vi "RIB Req - No Outputs.vi"(0 "Limits File Path":path, 5 "Results File Path":path, 11 "error in":errorcluster) -> (4 "Results Data Array":string[][](array[string]), 15 "error out":errorcluster)   [LabVIEW 2024]
doc: "Template test"
uses:
  <vilib>/addons/_JKI Toolkits/State Machine/_JKI_lib_State_Machine.llb/Select State(s)_err__jki_lib_state_machine.vi
  <vilib>/DAQmx/read.llb/DAQmx Read (Digital 1D Bool 1Chan 1Samp).vi
  <vilib>/addons/_JKI Toolkits/State Machine/_JKI_lib_State_Machine.llb/Select State(s)_bool__jki_lib_state_machine.vi
  <vilib>/addons/_JKI Toolkits/State Machine/_JKI_lib_State_Machine.llb/Periodic Trigger__ogtk__JKI-SM__jki_lib_state_machine.vi
  <userlib>/_OpenG.lib/file/file.llb/Strip Path Extension - String__ogtk.vi
  <vilib>/Utility/file.llb/Read Delimited Spreadsheet (string).vi
  <vilib>/DAQmx/miscellaneous.llb/DAQmx Fill In Error Info.vi
  <userlib>/_OpenG.lib/file/file.llb/openg_file.lvlib
  <userlib>/_OpenG.lib/appcontrol/appcontrol.llb/openg_application_control.lvlib
  <userlib>/_OpenG.lib/time/time.llb/openg_time.lvlib
  <vilib>/Utility/file.llb/Write Delimited Spreadsheet (string).vi
panel:
  in  "False":bool
  out "Results Data 3":string[](array[string])
  in  "task out":refnum<k21>
  out "Timeout":dbl(slide) scale=0.0..5.0
  in  "Exit":bool
  # "Both 15A and 5A Outputs are False"
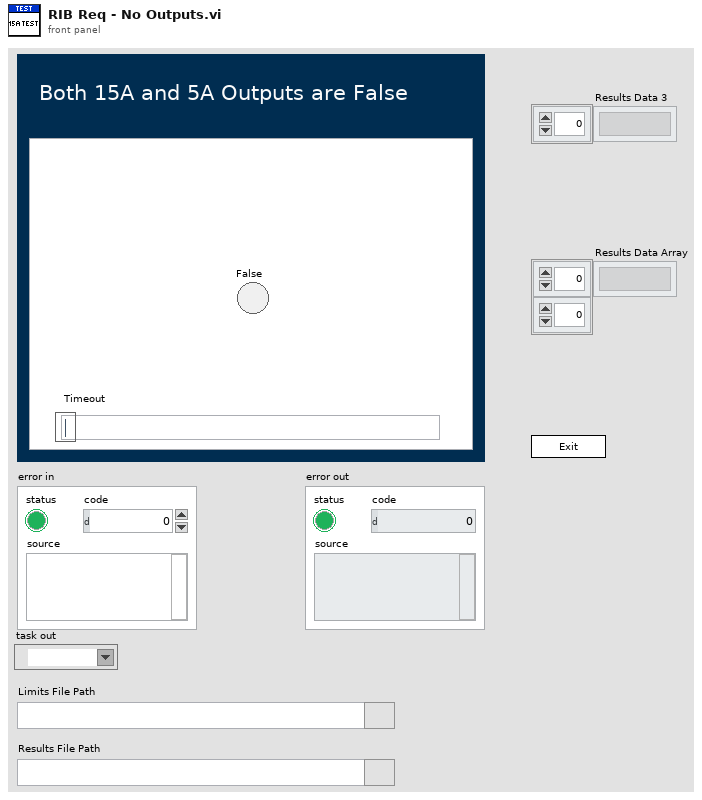
[diagram p1: front panel]
types:
  T1 = enum32{"Invalid", "Standard", "Closed", "Hidden", "Minimized", "Maximized"}
  T2 = enum32{"invalid app kind", "Development System", "Run Time System", "Student Edition", "Embedded LabVIEW", "Evaluation", "Custom"}
  T3 = typedef "FGV - Enum" = enum16{"Cleanup", "Get Data", "Simulator", "Open UDP", "Initialise DAQ", "Initialise I2C"}
  T4 = enum16{"Start Timer", "Get Time", "Pause", "Unpause"}
  T5 = cluster{"Core":cluster{"Current VI Reference":refnum<vi>, "Close Panel on Exit?":bool}, "Limits File Path":path, "Test Limits":string[][], "Results Data Array":string[][], "Results File Path":path, "task out":refnum<k21>, "False":bool}
  T6 = cluster{"Current VI Reference":refnum<vi>, "Close Panel on Exit?":bool}
  T7 = cluster{"[0]":bool, "[1]":bool, "[2]":bool, "[3]":bool, "[4]":bool, "[5]":bool, "[6]":bool, "[7]":bool, "[8]":bool}
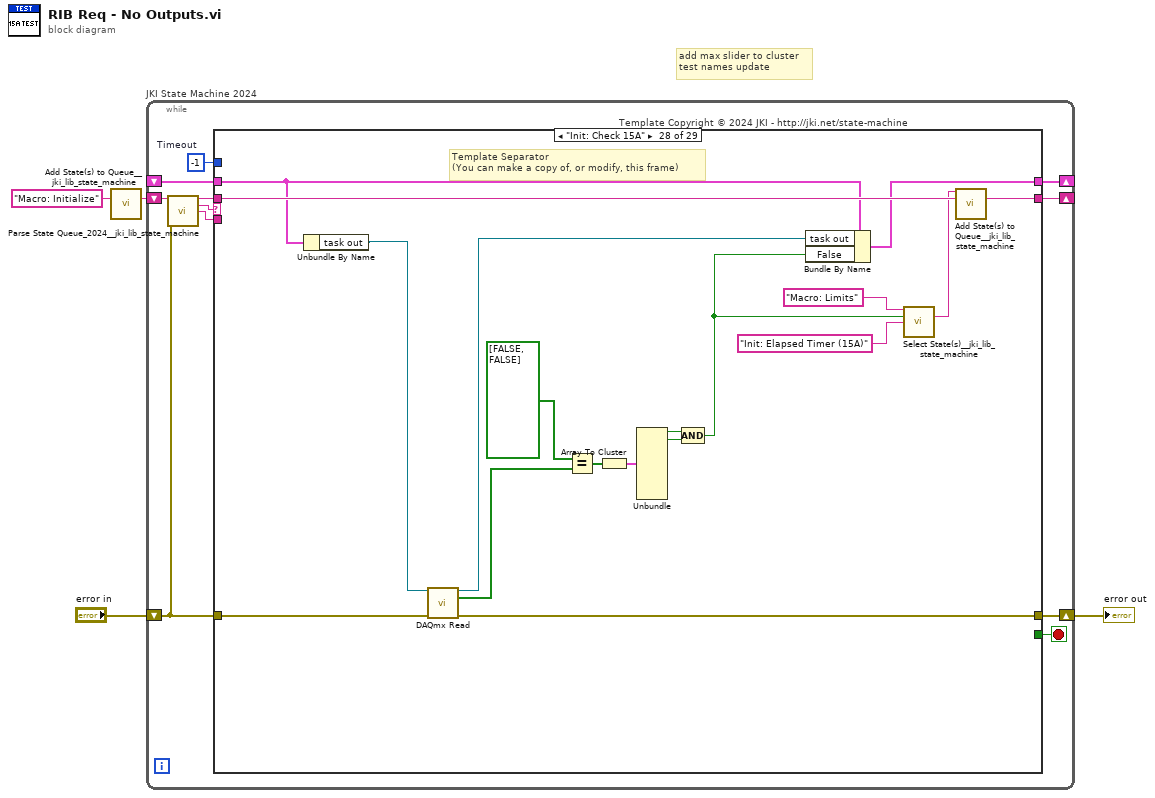
[diagram p0: block diagram]
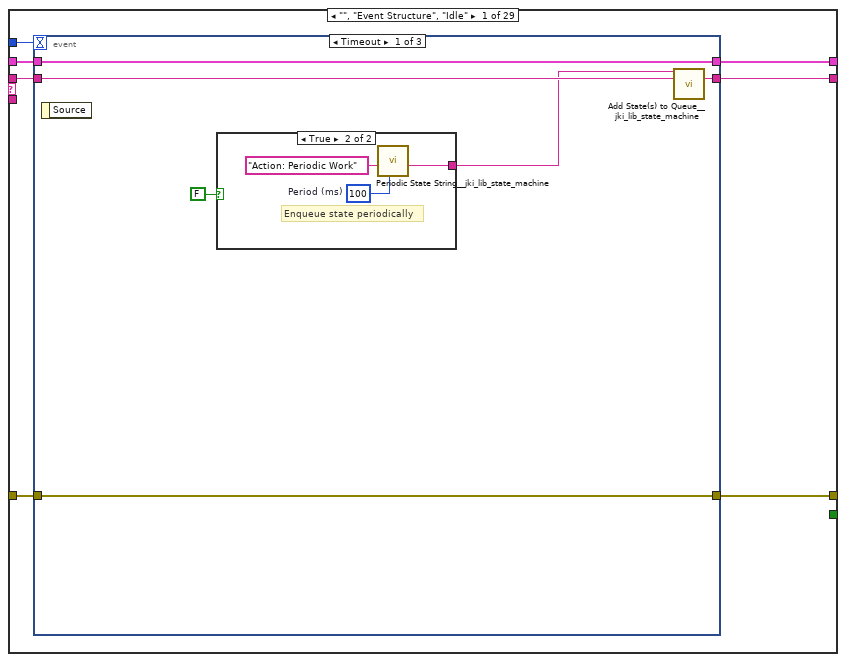
[diagram p2: hidden frame]
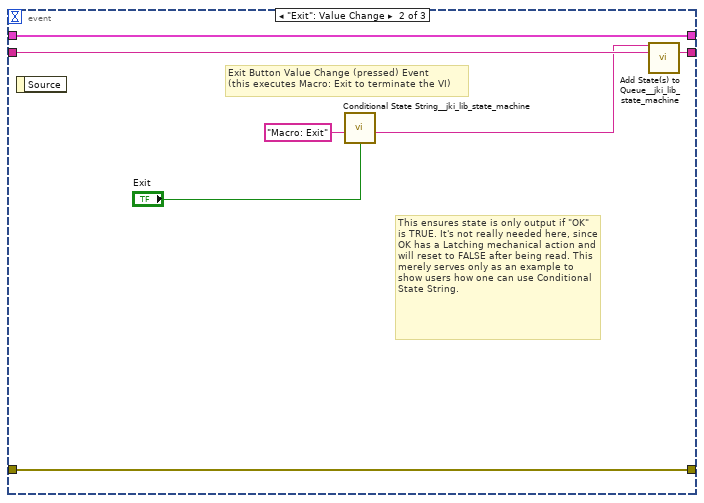
[diagram p4: hidden frame]
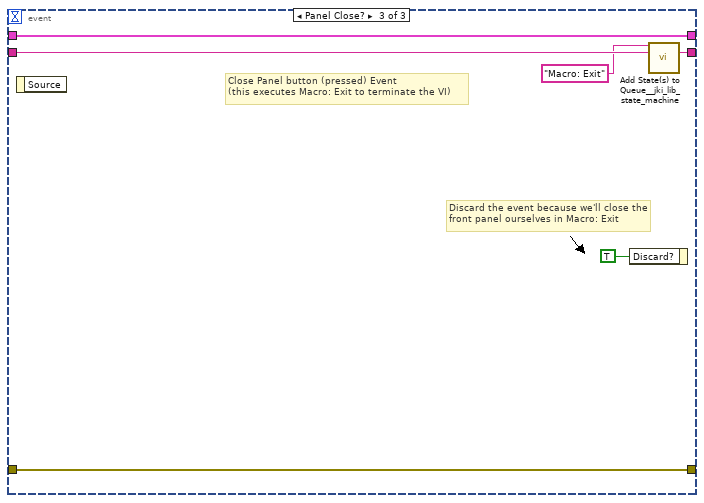
[diagram p5: hidden frame]
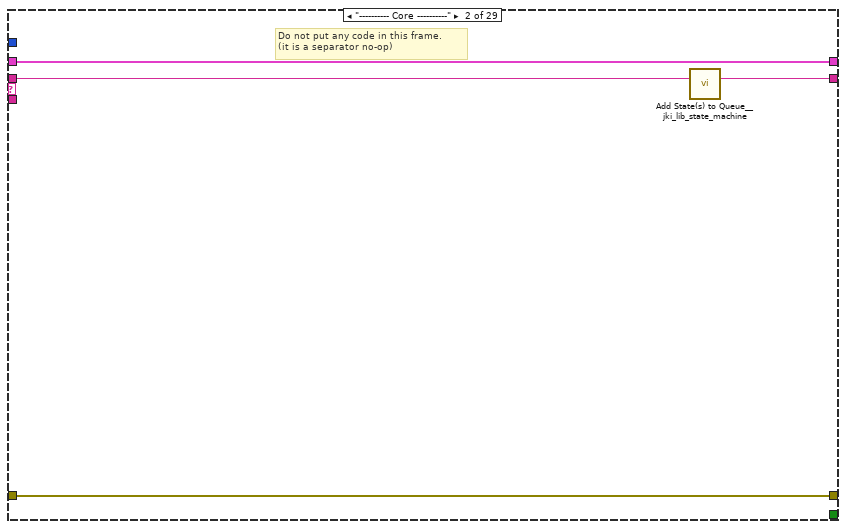
[diagram p6: hidden frame]
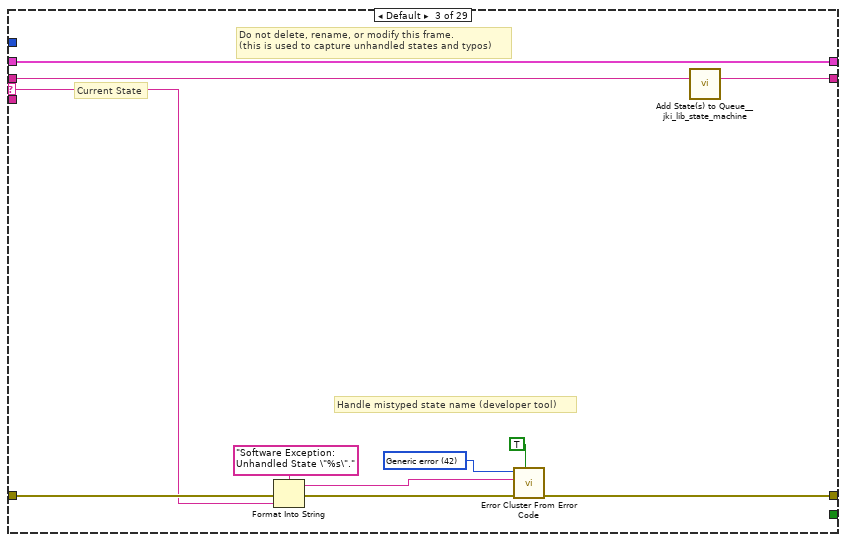
[diagram p7: hidden frame]
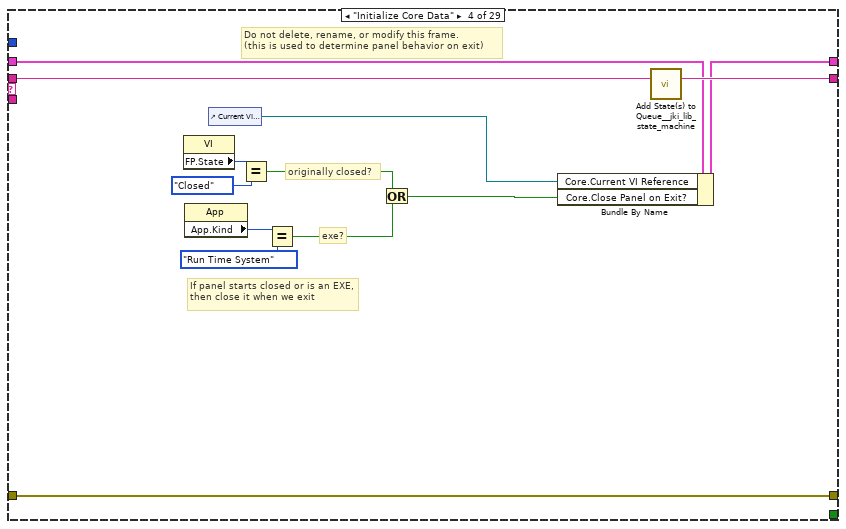
[diagram p8: hidden frame]
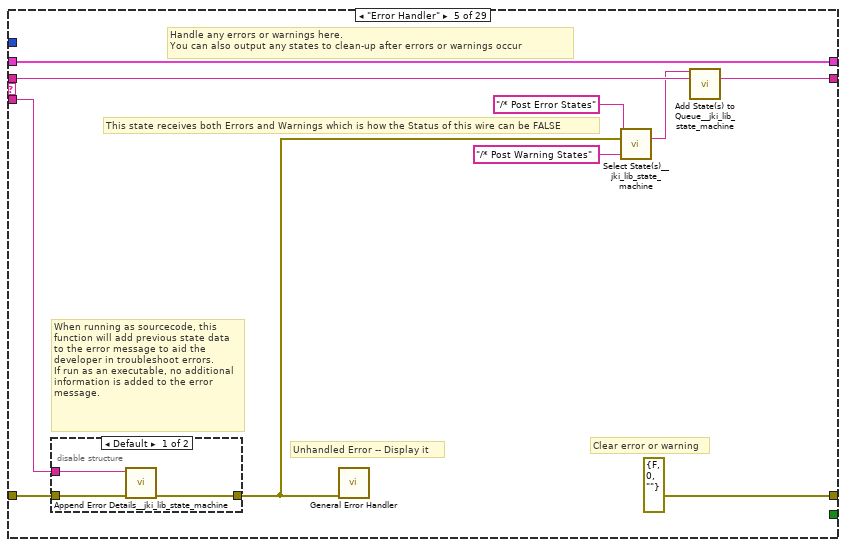
[diagram p9: hidden frame]
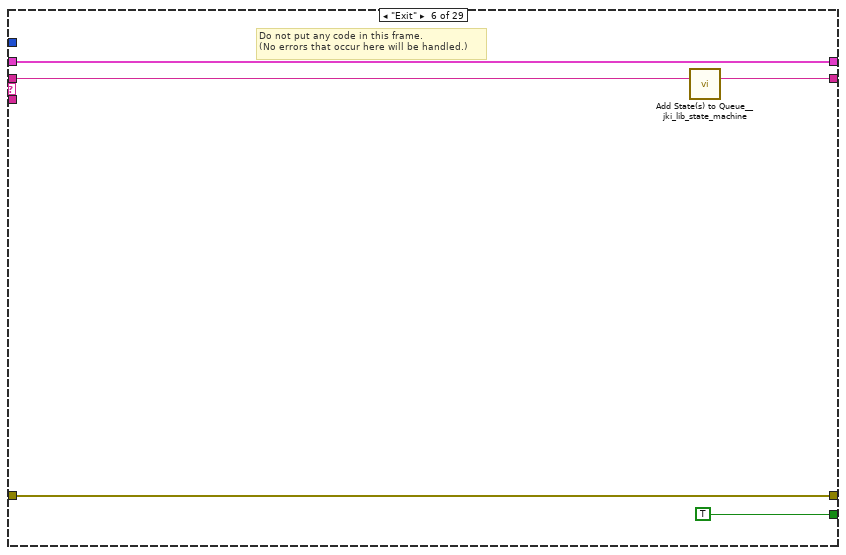
[diagram p11: hidden frame]
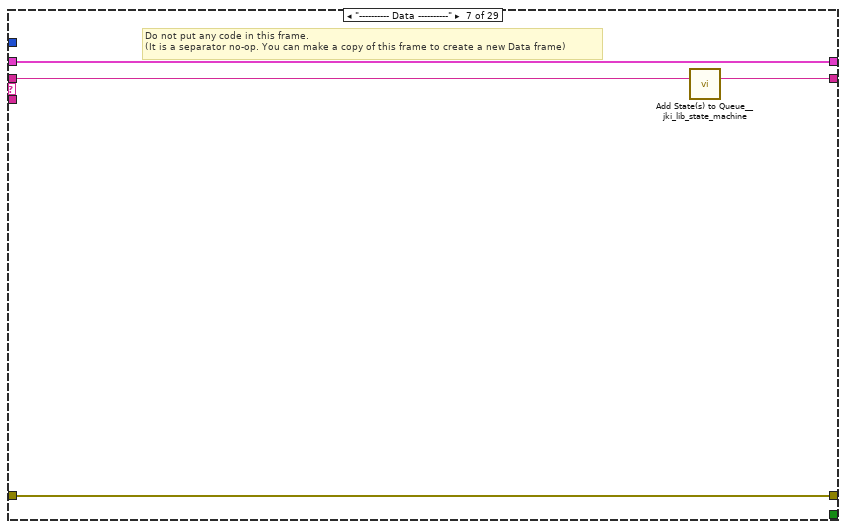
[diagram p12: hidden frame]
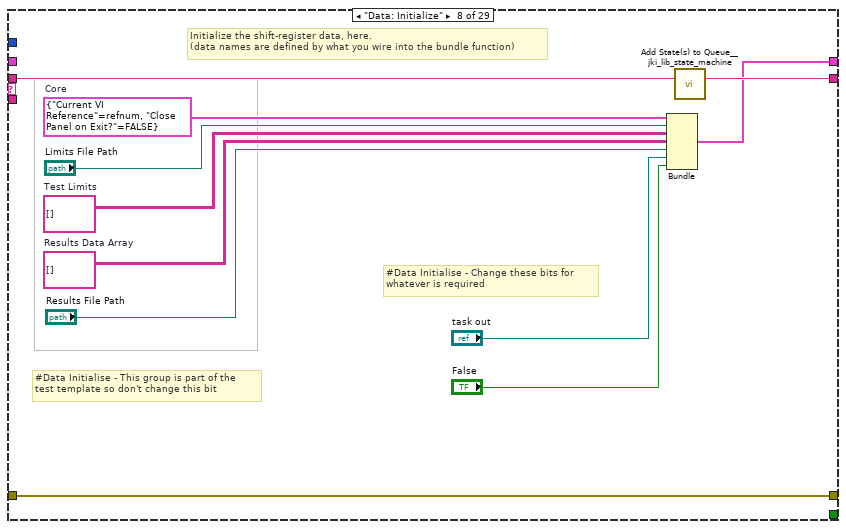
[diagram p13: hidden frame]
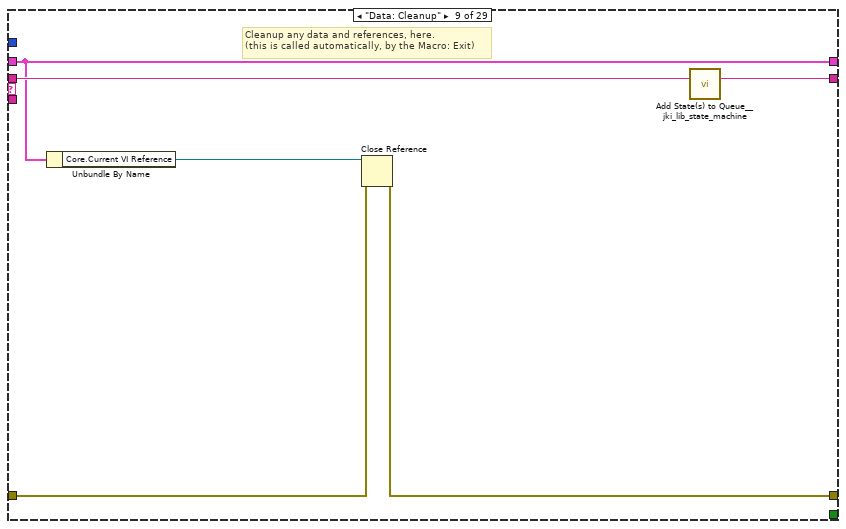
[diagram p14: hidden frame]
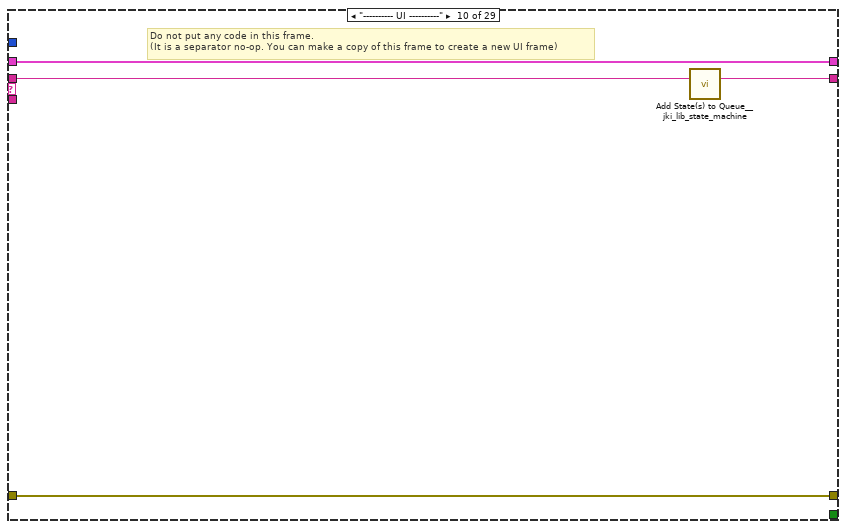
[diagram p15: hidden frame]
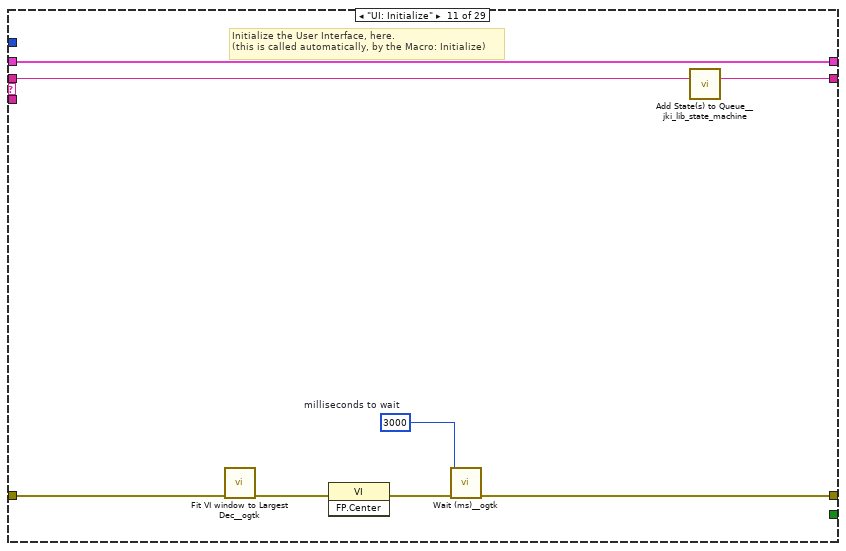
[diagram p16: hidden frame]
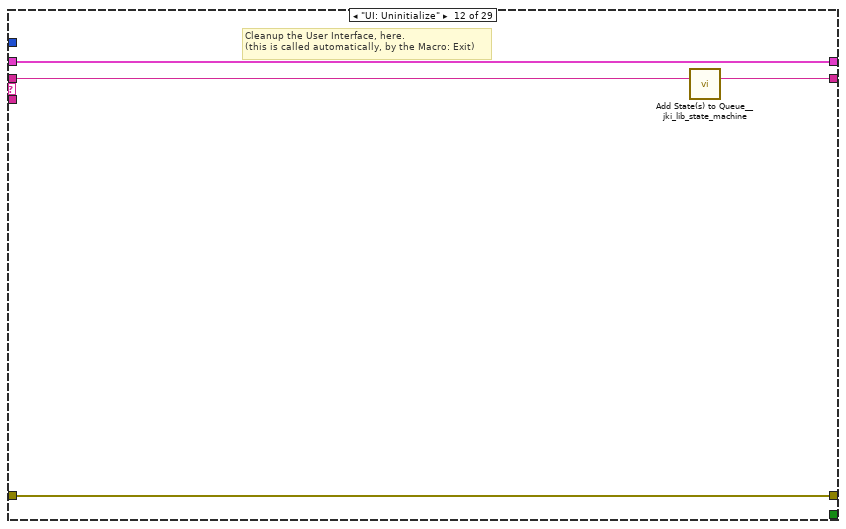
[diagram p17: hidden frame]
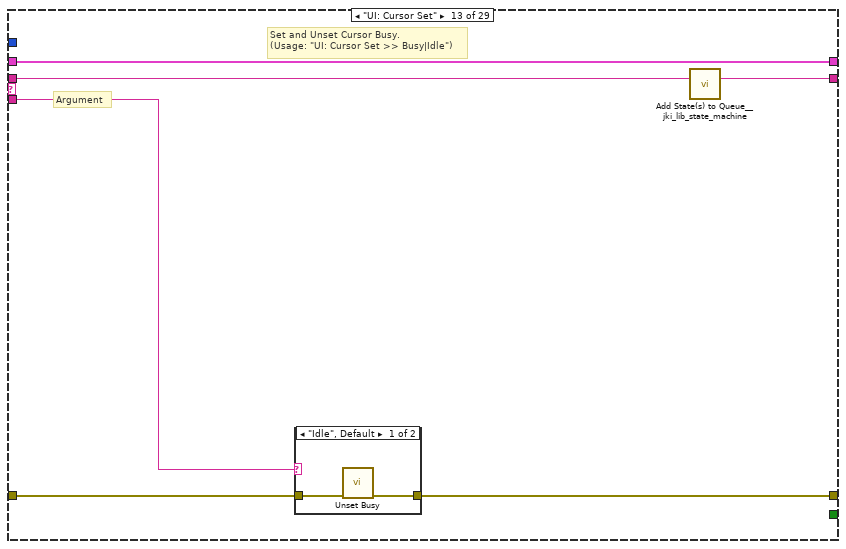
[diagram p18: hidden frame]
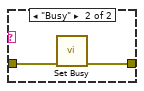
[diagram p19: hidden frame]
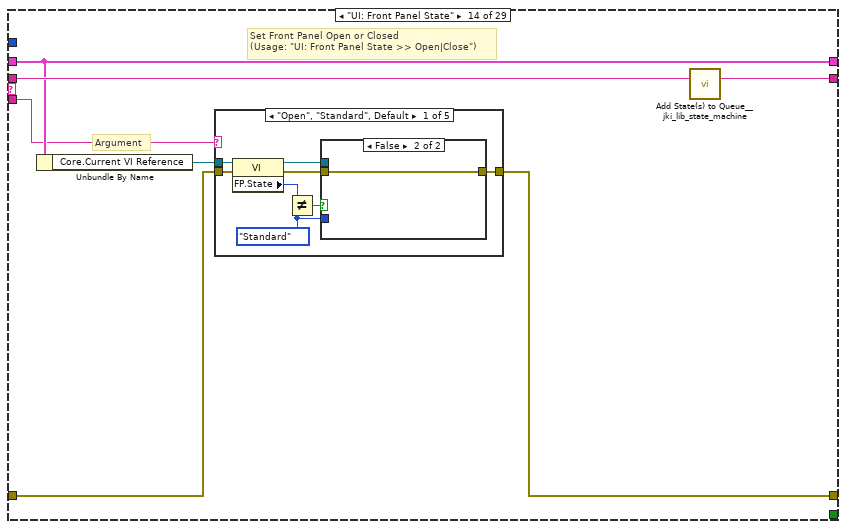
[diagram p20: hidden frame]
diagram:
  # "add max slider to cluster \ntest names update"
  n1 = call <vilib>:"Add State(s) to Queue__jki_lib_state_machine.vi"("State(s) in (\"\")"="Macro: Initialize") -> ("States Out"=w4:string)  [unwired: 14 in]
  n2 = while "JKI State Machine 2024" {
    shift-right: [w8] -> _
    shift-left: _ -> [w7]
    shift-right: [w11] -> w1
    shift-left: "error in" -> [w5]
    shift-right: [w10] -> _
    shift-left: w4 -> [w12]
    stop <- w9 stop-if-true
    w6 = -1  # Timeout
    # "Template Copyright © 2024 JKI - http://jki.net/state-machine"
    n3 = call <vilib>:"Parse State Queue_2024__jki_lib_state_machine.vi"("State Queue"=w12, "Error In (no error)"=w5) -> ("Remaining States"=w14:string, "Current State"=w15:string, "Arguments"=w13:string)  [unwired: 11 in]
    n4 = case shown="\"Init: Check 15A\"" w15 {
      selector: w15 -> [_ _ w49 _ _ _ _ _ _ _ _ _ _ _ _ _ _ _ _ _ _ _ _ _ _ _ _ _ _]
      tunnel: w14 -> [w22 w48 w53 w72 w82 w91 w95 w106 w112 w116 w124 w128 w134 w145 w214 w219 w224 w229 w238 w242 w255 w272 w276 w285 w289 w297 w308 w326 w338]
      tunnel: w13 -> [_ _ _ _ w77 _ _ _ _ _ _ _ w129 w139 _ _ _ _ _ _ _ _ _ _ _ _ _ _ _]
      tunnel: w7 -> [w20 w45 w51 w65 w79 w89 w92 _ w107 w113 w122 w126 w132 w141 w211 w216 w221 w226 w236 w239 w245 w264 w273 w281 w286 w295 w306 w322 w336]
      tunnel: [w19 w46 w55 w69 errorcluster {"status"=FALSE, "code"=0, "source"=""} ("error out") w88 w93 w103 w108 w114 w120 w125 w130 w142 w212 w217 w222 w227 w233 w240 w251 w269 w274 w283 w287 w292 w301 w312 w333] -> w11
      tunnel: w5 -> [w16 w46 w54 w69 w78 w88 w93 w103 w109 w114 w121 w125 w131 w143 w212 w217 w222 w227 w233 w240 w250 w268 w274 w282 w287 w291 w304 w313 w334]
      tunnel: [w21 w47 w52 w71 w81 w90 w94 w105 w111 w115 w123 w127 w133 w144 w213 w218 w223 w228 w237 w241 w254 w271 w275 w284 w288 w296 w307 w325 w337] -> w10
      tunnel: [_ _ _ _ _ TRUE _ _ _ _ _ _ _ _ _ _ _ _ _ _ _ _ _ _ _ _ _ _ _] -> w9
      tunnel: [w18 w45 w51 w70 w79 w89 w92 w104 w107 w113 w122 w126 w132 w141 w211 w216 w221 w226 w236 w239 w244 w263 w273 w281 w286 w294 w306 w321 w336] -> w8
      tunnel: w6 -> [w17 _ _ _ _ _ _ _ _ _ _ _ _ _ _ _ _ _ _ _ _ _ _ _ _ _ _ _ _]
      frame "", "Event Structure", "Idle" {
        n5 = event shown="[0] Timeout" {
          selector: _ -> [_ _ _]
          dyn-events: _ -> [_ _ _]
          timeout: w17 -> [_ _ _]
          tunnel: w22 -> [w28 w38 w44]
          tunnel: [w27 w37 w43] -> w21
          tunnel: w20 -> [w25 w35 w41]
          tunnel: [w26 w36 w42] -> w19
          tunnel: w16 -> [w26 w36 w42]
          tunnel: [w25 w35 w41] -> w18
          event Timeout {
            n6 = event-data() -> ()  [unwired: 1 in, 1 out]
            n7 = case shown="True" FALSE {
              tunnel: [_ w31] -> w24
              frame False {
              }
              frame True {
                w29 = u32 100  # Period (ms)
                # "Enqueue state periodically"
                n8 = call <vilib>:"Periodic State String__jki_lib_state_machine.vi"("Period (ms)"=w29, "State"="Action: Periodic Work") -> ("State Out"=w31:string)  [unwired: 9 in]
              }
            }
            n9 = call <vilib>:"Add State(s) to Queue__jki_lib_state_machine.vi"("State(s) in Front (\"\")"=w24, "State(s) in (\"\")"=w28) -> ("States Out"=w27:string)  [unwired: 13 in]
          }
          event "Exit": Value Change {
            # "This ensures state is only output if \"OK\" is TRUE. It's not really needed here, since OK has a Latching mechanical action and will reset to FALSE after being read. This merely serves only as an example to show users how one can use Conditional State String."
            # "Exit Button Value Change (pressed) Event\n(this executes Macro: Exit to terminate the VI)"
            n10 = event-data() -> ()  [unwired: 1 in, 1 out]
            n11 = call <vilib>:"Conditional State String__jki_lib_state_machine.vi"("Do State(s)?"="Exit", "State"="Macro: Exit") -> ("State Out"=w32:string)  [unwired: 7 in]
            n12 = call <vilib>:"Add State(s) to Queue__jki_lib_state_machine.vi"("State(s) in Front (\"\")"=w32, "State(s) in (\"\")"=w38) -> ("States Out"=w37:string)  [unwired: 13 in]
          }
          event Panel Close? {
            # "Discard the event because we'll close the front panel ourselves in Macro: Exit"
            # "Close Panel button (pressed) Event\n(this executes Macro: Exit to terminate the VI)"
            n13 = event-data() -> ()  [unwired: 1 in, 1 out]
            n14 = event-data("Discard?"=TRUE) -> ()  [unwired: 1 in, 1 out]
            n15 = call <vilib>:"Add State(s) to Queue__jki_lib_state_machine.vi"("State(s) in Front (\"\")"="Macro: Exit", "State(s) in (\"\")"=w44) -> ("States Out"=w43:string)  [unwired: 13 in]
          }
        }
      }
      frame "---------- Core ----------" {
        # "Do not put any code in this frame.\n(it is a separator no-op)"
        n16 = call <vilib>:"Add State(s) to Queue__jki_lib_state_machine.vi"("State(s) in (\"\")"=w48) -> ("States Out"=w47:string)  [unwired: 14 in]
      }
      frame Default {
        w58 = 42 items=["No error", "Argument error", "Memory is full", "Out of zone", "End of file", "File already open", "Generic file I/O error", "File not found", "File permission error", "Disk is full", "Duplicate path", "Too many files open", "System feature not enabled", "Resource file not found", "Cannot add resource", "Resource not found", "Image not found", "Image memory error", "Pen does not exist", "Config type invalid", "Config token not found", "Config parse error", "Config memory error", "Bad external code format", "Bad external code offset", "External code not present", "Null window", "Destroy window error", "Null menu", "Print aborted", "Bad print record", "Print driver error", "Windows error during printing", "Memory error during printing", "Print dialog error", "Generic print error", "Invalid device refnum", "Device not found", "Device parameter error", "Device unit error", "Cannot open device", "Device call aborted", "Generic error", "Cancelled by user", "Object ID too low", "Object ID too high", "Object not in heap", "Unknown heap", "Unknown object (invalid DefProc)", "Unknown object (DefProc not in table)", "Message out of range", "Invalid (null) method", "Unknown message", "Manager call not supported", "Bad address", "Network operation in progress", "Network operation timed out", "Connection is busy", "Network attribute not supported", "Network error", "Address in use", "System out of memory", "Connection aborted", "Connection refused", "Not connected", "Already connected", "Connection closed", "Initialization error (interapplication manager)", "Bad occurrence", "Wait on unbound occurrence handler", "Occurrence queue overflow", "Datalog type conflict", "Unused", "Unrecognized type (interapplication manager)", "Memory corrupt", "Failed to make temporary DLL", "Old CIN version", "Drag socket not found", "Failed to load drop-object", "Failed to register OLE object", "Failed to release OLE object", "Format specifier type mismatch", "Unknown format specifier", "Too few format specifiers", "Too many format specifiers", "Scan failed", "Newer CIN version", "Error converting to variant", "Runtime menu error", "Password tampered", "Variant attribute not found", "Incompatible variant data type", "Event data is not available", "Event Store is not present", "Occurrence is not found", "Event Queue is not created", "Event info is not available", "Refnum passed is NULL", "Error retrieving Class GUID", "Error retrieving CoClass GUID", "Error retrieving TypeLib GUID.", "Bad built application magic bytes.", "Specific driver is different from the specific driver associated with the Logical Name.", "There is no session opened to the class driver.", "Max Error", "MAX - Error with config objects", "MAX - Error loading configuration", "MAX - Group not supported"]
        # "Current State"
        # "Do not delete, rename, or modify this frame.\n(this is used to capture unhandled states and typos)"
        # "Handle mistyped state name (developer tool)"
        n17 = Format Into String(format string="Software Exception: Unhandled State \"%s\"." ("message"), error in=w54, w49) -> (resulting string=w57:string, error out=w56:errorcluster)  [unwired: 1 in]
        n18 = call <vilib>:"Error Cluster From Error Code.vi"("show call chain? (False)"=TRUE, "error in (no error)"=w56, "error message (\"\")"=w57, "error code (0)"=w58) -> ("error out"=w55:errorcluster)  [unwired: 5 in]
        n19 = call <vilib>:"Add State(s) to Queue__jki_lib_state_machine.vi"("State(s) in (\"\")"=w53) -> ("States Out"=w52:string)  [unwired: 14 in]
      }
      frame "Initialize Core Data" {
        # "Do not delete, rename, or modify this frame.\n(this is used to determine panel behavior on exit)"
        # "originally closed?"
        # "exe?"
        # "If panel starts closed or is an EXE, then close it when we exit"
        n20 = property class="VI"() -> ("FP.State"=w62:T1)  [unwired: 2 in, 2 out]
        n21 = property class="App"() -> ("App.Kind"=w68:T2)  [unwired: 2 in, 2 out]
        n22 = control-ref of="Current VI Reference"() -> (w63:refnum<vi>)
        n23 = Equal?(x=w62, y=T1."Closed" ("Front Panel Window:State")) -> (x = y?=w60:bool)
        n24 = Equal?(x=w68, y=T2."Run Time System" ("Application:Kind")) -> (x = y?=w66:bool)
        n25 = Or(x=w60, y=w66) -> (x .or. y?=w64:bool)
        n26 = Bundle By Name(cluster=w65, "Core.Current VI Reference"=w63, "Core.Close Panel on Exit?"=w64) -> (w70:T5)
        n27 = call <vilib>:"Add State(s) to Queue__jki_lib_state_machine.vi"("State(s) in (\"\")"=w72) -> ("States Out"=w71:string)  [unwired: 14 in]
      }
      frame "Error Handler" {
        # "When running as sourcecode, this function will add previous state data to the error message to aid the developer in troubleshoot errors.\nIf run as an executable, no additional information is added to the error message."
        # "This state receives both Errors and Warnings which is how the Status of this wire can be FALSE"
        # "Unhandled Error -- Display it"
        # "Handle any errors or warnings here.\nYou can also output any states to clean-up after errors or warnings occur"
        # "Clear error or warning"
        n28 = disable-structure shown="Default" {
          disable-tunnel: w78 -> [w85 w86]
          disable-tunnel: w77 -> [w84 _]
          disable-tunnel: [w83 w86] -> w76
          frame condition #0 (active) {
            n29 = call <vilib>:"Append Error Details__jki_lib_state_machine.vi"("error in (no error)"=w85, "Previous State and Argument(s)"=w84) -> ("error out"=w83:errorcluster)  [unwired: 9 in]
          }
          frame condition #1 {
          }
        }
        n30 = call <vilib>:"General Error Handler.vi"("error in (no error)"=w76) -> ()  [unwired: 10 in, 5 out]
        n31 = call-poly <vilib>:"Select State(s)__jki_lib_state_machine.vi"("State(s) if True (\"\")"="/* Post Error States", "Select"=w76, "State(s) if False (\"\")"="/* Post Warning States") -> ("States Out"=w74:string)  [unwired: 12 in]
        n32 = call <vilib>:"Add State(s) to Queue__jki_lib_state_machine.vi"("State(s) in Front (\"\")"=w74, "State(s) in (\"\")"=w82) -> ("States Out"=w81:string)  [unwired: 13 in]
      }
      frame "Exit" {
        # "Do not put any code in this frame.\n(No errors that occur here will be handled.)"
        n33 = call <vilib>:"Add State(s) to Queue__jki_lib_state_machine.vi"("State(s) in (\"\")"=w91) -> ("States Out"=w90:string)  [unwired: 14 in]
      }
      frame "---------- Data ----------" {
        # "Do not put any code in this frame.\n(It is a separator no-op. You can make a copy of this frame to create a new Data frame)"
        n34 = call <vilib>:"Add State(s) to Queue__jki_lib_state_machine.vi"("State(s) in (\"\")"=w95) -> ("States Out"=w94:string)  [unwired: 14 in]
      }
      frame "Data: Initialize" {
        w99 = string[][] []  # Results Data Array
        w100 = string[][] []  # Test Limits
        w102 = T6 {"Current VI Reference"=refnum, "Close Panel on Exit?"=FALSE}  # Core
        # "#Data Initialise - Change these bits for\nwhatever is required"
        # "#Data Initialise - This group is part of the\ntest template so don't change this bit"
        # "Initialize the shift-register data, here.\n(data names are defined by what you wire into the bundle function)"
        n35 = Bundle("Core"=w102, "Limits File Path"="Limits File Path", "Test Limits"=w100, "Results Data Array"=w99, "Results File Path"="Results File Path", "task out"="task out", "False"="False") -> (w104:T5)  [unwired: 1 in]
        n36 = call <vilib>:"Add State(s) to Queue__jki_lib_state_machine.vi"("State(s) in (\"\")"=w106) -> ("States Out"=w105:string)  [unwired: 14 in]
      }
      frame "Data: Cleanup" {
        # "Cleanup any data and references, here.\n(this is called automatically, by the Macro: Exit)"
        n37 = Unbundle By Name(w107) -> ("Core.Current VI Reference"=w110:refnum<vi>)
        n38 = Close Reference(reference=w110, error in (no error)=w109) -> (error out=w108:errorcluster)
        n39 = call <vilib>:"Add State(s) to Queue__jki_lib_state_machine.vi"("State(s) in (\"\")"=w112) -> ("States Out"=w111:string)  [unwired: 14 in]
      }
      frame "---------- UI ----------" {
        # "Do not put any code in this frame.\n(It is a separator no-op. You can make a copy of this frame to create a new UI frame)"
        n40 = call <vilib>:"Add State(s) to Queue__jki_lib_state_machine.vi"("State(s) in (\"\")"=w116) -> ("States Out"=w115:string)  [unwired: 14 in]
      }
      frame "UI: Initialize" {
        w119 = u32 3000  # milliseconds to wait
        # "Initialize the User Interface, here.\n(this is called automatically, by the Macro: Initialize)"
        n41 = call <userlib>:"Fit VI window to Largest Dec__ogtk.vi"("error in (no error)"=w121) -> ("error out"=w117:errorcluster)  [unwired: 5 in, 1 out]
        n42 = invoke class="VI" method="FP.Center"(error in=w117) -> (error out=w118:errorcluster)  [unwired: 2 in, 2 out]
        n43 = call <userlib>:"Wait (ms)__ogtk.vi"("error in (no error)"=w118, "milliseconds to wait"=w119) -> ("error out"=w120:errorcluster)  [unwired: 8 in, 1 out]
        n44 = call <vilib>:"Add State(s) to Queue__jki_lib_state_machine.vi"("State(s) in (\"\")"=w124) -> ("States Out"=w123:string)  [unwired: 14 in]
      }
      frame "UI: Uninitialize" {
        # "Cleanup the User Interface, here.\n(this is called automatically, by the Macro: Exit)"
        n45 = call <vilib>:"Add State(s) to Queue__jki_lib_state_machine.vi"("State(s) in (\"\")"=w128) -> ("States Out"=w127:string)  [unwired: 14 in]
      }
      frame "UI: Cursor Set" {
        # "Argument"
        # "Set and Unset Cursor Busy.\n(Usage: \"UI: Cursor Set >> Busy|Idle\")"
        n46 = case shown="\"Idle\", Default" w129 {
          tunnel: w131 -> [w136 w138]
          tunnel: [w135 w137] -> w130
          frame "Idle", Default {
            n47 = call <vilib>:"Unset Busy.vi"("error in (no error)"=w136) -> ("error out"=w135:errorcluster)  [unwired: 10 in]
          }
          frame "Busy" {
            n48 = call <vilib>:"Set Busy.vi"("error in (no error)"=w138) -> ("error out"=w137:errorcluster)  [unwired: 9 in, 1 out]
          }
        }
        n49 = call <vilib>:"Add State(s) to Queue__jki_lib_state_machine.vi"("State(s) in (\"\")"=w134) -> ("States Out"=w133:string)  [unwired: 14 in]
      }
      frame "UI: Front Panel State" {
        # "Argument"
        # "Set Front Panel Open or Closed\n(Usage: \"UI: Front Panel State >> Open|Close\")"
        n50 = Unbundle By Name(w141) -> ("Core.Current VI Reference"=w140:refnum<vi>)
        n51 = case shown="\"Open\", \"Standard\", Default" w139 {
          tunnel: w143 -> [w151 w166 w177 w190 w203]
          tunnel: [w153 w167 w179 w192 w205] -> w142
          tunnel: w140 -> [w152 w164 w178 w191 w204]
          frame "Open", "Standard", Default {
            w146 = T1."Standard" ("State")
            n52 = property class="VI"(reference=w152, error in=w151) -> (reference out=w149:refnum<vi>, error out=w150:errorcluster, "FP.State"=w148:T1)
            n53 = Not Equal?(x=w148, y=w146) -> (x != y?=w147:bool)
            n54 = case shown="False" w147 {
              tunnel: [w157 w159] -> w153
              tunnel: w150 -> [w156 w159]
              tunnel: w149 -> [w155 _]
              tunnel: w146 -> [w154 _]
              frame True {
                n55 = invoke class="VI" method="FP.Open"(reference=w155, error in=w156, "Activate"=TRUE, "State"=w154) -> (error out=w157:errorcluster)  [unwired: 1 in, 4 out]
              }
              frame False {
              }
            }
          }
          frame "Close", "Closed" {
            n56 = property class="VI"(reference=w164, error in=w166) -> (reference out=w163:refnum<vi>, error out=w165:errorcluster, "FP.State"=w161:T1)
            n57 = Not Equal?(x=w161, y=T1."Closed" ("Front Panel Window:State")) -> (x != y?=w160:bool)
            n58 = case shown="True" w160 {
              tunnel: [w168 w171] -> w167
              tunnel: w165 -> [w168 w170]
              tunnel: w163 -> [_ w169]
              frame False {
              }
              frame True {
                n59 = invoke class="VI" method="FP.Close"(reference=w169, error in=w170) -> (error out=w171:errorcluster)  [unwired: 1 in, 2 out]
              }
            }
          }
          frame "Hidden", "Hide" {
            w172 = T1."Hidden" ("State")
            n60 = property class="VI"(reference=w178, error in=w177) -> (reference out=w175:refnum<vi>, error out=w176:errorcluster, "FP.State"=w174:T1)
            n61 = Not Equal?(x=w174, y=w172) -> (x != y?=w173:bool)
            n62 = case shown="True" w173 {
              tunnel: [w183 w184] -> w179
              tunnel: w176 -> [w182 w184]
              tunnel: w175 -> [w181 _]
              tunnel: w172 -> [w180 _]
              frame True {
                n63 = invoke class="VI" method="FP.Open"(reference=w181, error in=w182, "State"=w180) -> (error out=w183:errorcluster)  [unwired: 2 in, 4 out]
              }
              frame False {
              }
            }
          }
          frame "Minimize", "Minimized" {
            w185 = T1."Minimized" ("State")
            n64 = property class="VI"(reference=w191, error in=w190) -> (reference out=w188:refnum<vi>, error out=w189:errorcluster, "FP.State"=w187:T1)
            n65 = Not Equal?(x=w187, y=w185) -> (x != y?=w186:bool)
            n66 = case shown="True" w186 {
              tunnel: [w196 w197] -> w192
              tunnel: w189 -> [w195 w197]
              tunnel: w188 -> [w194 _]
              tunnel: w185 -> [w193 _]
              frame True {
                n67 = invoke class="VI" method="FP.Open"(reference=w194, error in=w195, "State"=w193) -> (error out=w196:errorcluster)  [unwired: 2 in, 4 out]
              }
              frame False {
              }
            }
          }
          frame "Maximize", "Maximized" {
            w198 = T1."Maximized" ("State")
            n68 = property class="VI"(reference=w204, error in=w203) -> (reference out=w201:refnum<vi>, error out=w202:errorcluster, "FP.State"=w200:T1)
            n69 = Not Equal?(x=w200, y=w198) -> (x != y?=w199:bool)
            n70 = case shown="True" w199 {
              tunnel: [w209 w210] -> w205
              tunnel: w202 -> [w208 w210]
              tunnel: w201 -> [w207 _]
              tunnel: w198 -> [w206 _]
              frame True {
                n71 = invoke class="VI" method="FP.Open"(reference=w207, error in=w208, "State"=w206) -> (error out=w209:errorcluster)  [unwired: 2 in, 4 out]
              }
              frame False {
              }
            }
          }
        }
        n72 = call <vilib>:"Add State(s) to Queue__jki_lib_state_machine.vi"("State(s) in (\"\")"=w145) -> ("States Out"=w144:string)  [unwired: 14 in]
      }
      frame "---------- Macro ----------" {
        # "Do not put any code in this frame.\n(It is a separator no-op. You can make a copy of this frame to create a new Macro frame)"
        n73 = call <vilib>:"Add State(s) to Queue__jki_lib_state_machine.vi"("State(s) in (\"\")"=w214) -> ("States Out"=w213:string)  [unwired: 14 in]
      }
      frame "Macro: Initialize" {
        # "Initialization Macro\n(This is called once, when the VI starts)"
        n74 = call <vilib>:"Add State(s) to Queue__jki_lib_state_machine.vi"("State(s) in Front (\"\")"="Data: Initialize\nInitialize Core Data\nUI: Initialize\nUI: Front Panel State >> Open\nMacro: Test", "State(s) in (\"\")"=w219) -> ("States Out"=w218:string)  [unwired: 13 in]
      }
      frame "Macro: Test" {
        # "#Test Macro - Add the sequence \nfor measurments and limits testing here"
        n75 = call <vilib>:"Add State(s) to Queue__jki_lib_state_machine.vi"("State(s) in Front (\"\")"="Limits Test: Read Limits File\nInit: I2C Open\nInit: Start Timer (15A)", "State(s) in (\"\")"=w224) -> ("States Out"=w223:string)  [unwired: 13 in]
      }
      frame "Macro: Limits" {
        # "Do not put any code in this frame.\n(It is a separator no-op. You can make a copy of this frame to create a new Macro frame)"
        n76 = call <vilib>:"Add State(s) to Queue__jki_lib_state_machine.vi"("State(s) in Front (\"\")"="Limits Test: 5A Read Test\nResults Data: Write Results Data\nMacro: Exit", "State(s) in (\"\")"=w229) -> ("States Out"=w228:string)  [unwired: 13 in]
      }
      frame "Macro: Exit" {
        # "Exit Macro\n(This is called once, when the VI exits)"
        n77 = Unbundle By Name(w236) -> ("Core.Close Panel on Exit?"=w231:bool)
        n78 = call <vilib>:"Conditional State String__jki_lib_state_machine.vi"("Do State(s)?"=w231, "State"="UI: Front Panel State >> Close") -> ("State Out"=w230:string)  [unwired: 7 in]
        n79 = call <vilib>:"Add State(s) to Queue__jki_lib_state_machine.vi"("State(s) in (\"\")"=w230, "State(s) at Back (\"\")"="UI: Uninitialize\nData: Cleanup\nExit") -> ("States Out"=w234:string)  [unwired: 13 in]
        n80 = call <vilib>:"Add State(s) to Queue__jki_lib_state_machine.vi"("State(s) in Front (\"\")"=w234, "State(s) in (\"\")"=w238) -> ("States Out"=w237:string)  [unwired: 13 in]
      }
      frame "---------- Limits Test ----------" {
        # "Template Separator\n(You can make a copy of, or modify, this frame)"
        n81 = call <vilib>:"Add State(s) to Queue__jki_lib_state_machine.vi"("State(s) in (\"\")"=w242) -> ("States Out"=w241:string)  [unwired: 14 in]
      }
      frame "Limits Test: Read Limits File" {
        w248 = ","  # delimiter (\t)
        n82 = Unbundle By Name(w245) -> ("Limits File Path"=w249:path)
        n83 = Current VI's Path "Test Case Path"() -> (path=w253:path)
        n84 = call-poly <vilib>:"Read Delimited Spreadsheet.vi"("file path (dialog if empty)"=w249, "error in (no error)"=w250, "delimiter (\\t)"=w248) -> ("all rows"=w246:string[][], "error out"=w251:errorcluster)  [unwired: 7 in, 4 out]
        n85 = Strip Path(path=w253) -> (name=w252:string)  [unwired: 1 out]
        n86 = call-poly <userlib>:"Strip Path Extension__ogtk.vi"("path"=w252) -> ("root"=w247:string)  [unwired: 1 out]
        n87 = for {
          tunnel: w247 -> [w259]
          tunnel: w246 -> [w257] mode=indexing
          tunnel: [w257] -> w243 mode=indexing if=w256
          n88 = Index Array(array=w257) -> (element=w258:string)  [unwired: 1 in]
          n89 = Equal?(x=w259, y=w258) -> (x = y?=w256:bool)
        }
        n90 = Bundle By Name(cluster=w245, "Test Limits"=w243) -> (w244:T5)
        n91 = call <vilib>:"Add State(s) to Queue__jki_lib_state_machine.vi"("State(s) in (\"\")"=w255) -> ("States Out"=w254:string)  [unwired: 14 in]
      }
      frame "Limits Test: 5A Read Test" {
        w265 = "False Read Test"  # Sub Test Name
        # "UDP Read Test = if equal to F0 = pass else fail"
        # "#Limits Testing - Add the sub test name for\ntest included in limits file"
        n92 = Unbundle By Name(w264) -> ("Results Data Array"=w262:string[][])
        n93 = Unbundle By Name(w264) -> ("Test Limits"=w266:string[][], "False"=w270:bool)
        n94 = To Variant(anything=w270) -> (Variant=w267:variant)
        n95 = call "Process Results.vi"("error in (no error)"=w268, "Measurement"=w267, "Test Limits"=w266, "Sub Test Name"=w265) -> ("error out"=w269:errorcluster, "Results Data"=w260:string[])  [unwired: 6 in]
        "Results Data 3" <- w260
        n96 = Build Array (concatenate)(w262, w260) -> (w261:string[][])
        n97 = Bundle By Name(cluster=w264, "Results Data Array"=w261) -> (w263:T5)
        n98 = call <vilib>:"Add State(s) to Queue__jki_lib_state_machine.vi"("State(s) in (\"\")"=w272) -> ("States Out"=w271:string)  [unwired: 14 in]
      }
      frame "---------- Results Data ----------" {
        # "Template Separator\n(You can make a copy of, or modify, this frame)"
        n99 = call <vilib>:"Add State(s) to Queue__jki_lib_state_machine.vi"("State(s) in (\"\")"=w276) -> ("States Out"=w275:string)  [unwired: 14 in]
      }
      frame "Results Data: Write Results Data" {
        w278 = ","  # delimiter (\t)
        w279 = TRUE  # append to file? (new file:F)
        n100 = Unbundle By Name(w281) -> ("Results File Path"=w280:path, "Results Data Array"=w277:string[][])
        "Results Data Array" <- w277
        n101 = call-poly <vilib>:"Write Delimited Spreadsheet.vi"("file path (dialog if empty)"=w280, "2D data"=w277, "append to file? (new file:F)"=w279, "error in (no error)"=w282, "delimiter (\\t)"=w278) -> ("error out"=w283:errorcluster)  [unwired: 9 in, 1 out]
        n102 = call <vilib>:"Add State(s) to Queue__jki_lib_state_machine.vi"("State(s) in (\"\")"=w285) -> ("States Out"=w284:string)  [unwired: 14 in]
      }
      frame "---------- Init ----------" {
        # "Template Separator\n(You can make a copy of, or modify, this frame)"
        n103 = call <vilib>:"Add State(s) to Queue__jki_lib_state_machine.vi"("State(s) in (\"\")"=w289) -> ("States Out"=w288:string)  [unwired: 14 in]
      }
      frame "Init: I2C Open" {
        # "Template Separator\n(You can make a copy of, or modify, this frame)"
        n104 = call "FGV - Initialise.vi"("Enum"=FGV_-_Enum."Get Data", "Error In"=w291) -> ("task out"=w290:refnum<k21>, "Error Out"=w292:errorcluster)  [unwired: 13 in, 3 out]
        n105 = Bundle By Name(cluster=w295, "task out"=w290) -> (w294:T5)
        n106 = call <vilib>:"Add State(s) to Queue__jki_lib_state_machine.vi"("State(s) in (\"\")"=w297) -> ("States Out"=w296:string)  [unwired: 14 in]
      }
      frame "Init: Start Timer (15A)" {
        # "Start 10 second timer"
        # "Template Separator\n(You can make a copy of, or modify, this frame)"
        n107 = call "Timer.vi"("error in (no error)"=w304, "Enum"=T4."Start Timer") -> ("error out"=w302:errorcluster)  [unwired: 6 in, 3 out]
        n108 = property on="Timeout" class="Slide (strict)"(error in=w302, "Value"=0.0 ("Horizontal Pointer Slide"), "Scale.Maximum"=5.0 ("Target Time"), "Scale.Minimum"=0.0 ("Scale.Range:Minimum")) -> (error out=w301:errorcluster)  [unwired: 1 in, 1 out]
        n109 = call <vilib>:"Add State(s) to Queue__jki_lib_state_machine.vi"("State(s) in Front (\"\")"="Init: Check 15A" ("State(s) in Front (\"\")"), "State(s) in (\"\")"=w308) -> ("States Out"=w307:string)  [unwired: 13 in]
      }
      frame "Init: Check 15A" {
        # "Template Separator\n(You can make a copy of, or modify, this frame)"
        n110 = Unbundle By Name(w322) -> ("task out"=w314:refnum<k21>)
        n111 = call-poly <vilib>:"DAQmx Read.vi"("task/channels in"=w314, "error in"=w313) -> ("task out"=w309:refnum<k21>, "data"=w320:bool[], "error out"=w312:errorcluster)  [unwired: 11 in]
        n112 = Equal?(x=bool[] [FALSE, FALSE], y=w320) -> (x = y?=w316:bool[])
        n113 = Array To Cluster(array=w316) -> (cluster=w317:T7)
        n114 = Unbundle(w317) -> ("[0]"=w318:bool, "[1]"=w319:bool)  [unwired: 7 out]
        n115 = Compound Arithmetic op=AND(w318, w319) -> (w310:bool)
        n116 = Bundle By Name(cluster=w322, "task out"=w309, "False"=w310) -> (w321:T5)
        n117 = call-poly <vilib>:"Select State(s)__jki_lib_state_machine.vi"("State(s) if True (\"\")"="Macro: Limits" ("State(s) if True (\"\")"), "Select"=w310, "State(s) if False (\"\")"="Init: Elapsed Timer (15A)" ("State(s) if False (\"\")")) -> ("States Out"=w323:string)  [unwired: 12 in]
        n118 = call <vilib>:"Add State(s) to Queue__jki_lib_state_machine.vi"("State(s) in Front (\"\")"=w323, "State(s) in (\"\")"=w326) -> ("States Out"=w325:string)  [unwired: 13 in]
      }
      frame "Init: Elapsed Timer (15A)" {
        # "check if timer elased - if TRUE end test if FALSE read UDP again."
        # "Template Separator\n(You can make a copy of, or modify, this frame)"
        n119 = call "Timer.vi"("error in (no error)"=w334, "Target Time"=5.0, "Enum"=T4."Get Time") -> ("error out"=w333:errorcluster, "Time Elapsed?"=w330:bool, "Elapsed Time"=→"Timeout":dbl)  [unwired: 5 in, 1 out]
        n120 = call-poly <vilib>:"Select State(s)__jki_lib_state_machine.vi"("State(s) if True (\"\")"="Macro: Limits" ("State(s) if True (\"\")"), "Select"=w330, "State(s) if False (\"\")"="Init: Check 15A" ("State(s) if False (\"\")")) -> ("States Out"=w329:string)  [unwired: 12 in]
        n121 = call <vilib>:"Add State(s) to Queue__jki_lib_state_machine.vi"("State(s) in Front (\"\")"=w329, "State(s) in (\"\")"=w338) -> ("States Out"=w337:string)  [unwired: 13 in]
      }
    }
  }
  "error out" <- w1
